vi "main.vi"() -> ()   [LabVIEW 2023]
uses:
  CONTROLS/states.ctl
panel:
  out "Meldung":string
  out "Enum":T1
  in  "stop":bool
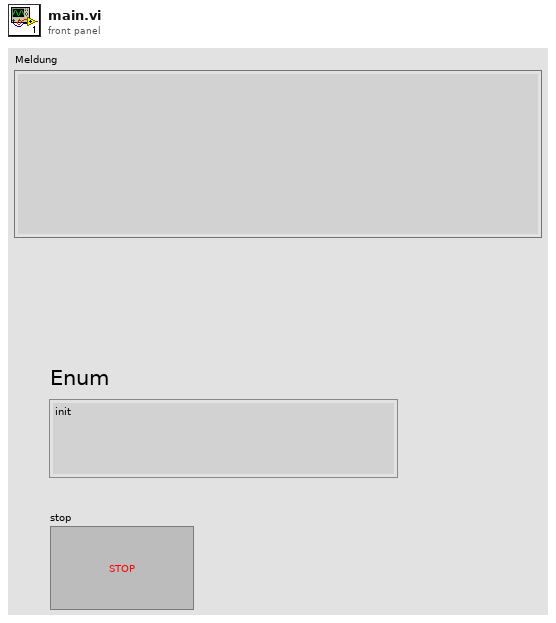
[diagram p1: front panel]
types:
  T1 = typedef "states.ctl" = enum16{"init", "read", "write", "Kundeneingabe", "Betonauswahl", "Bezahlprozeß", "Rechnung", "Zudaten mit Gewichtmessung", "Stop"}
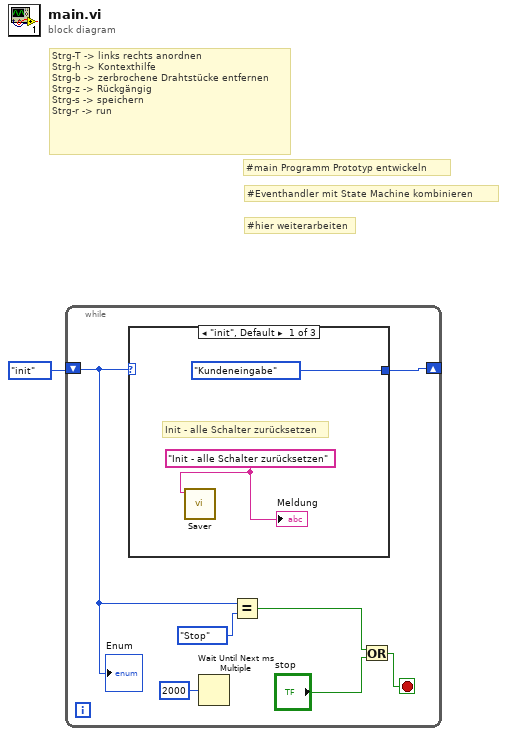
[diagram p0: block diagram]
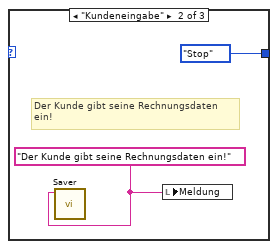
[diagram p2: hidden frame]
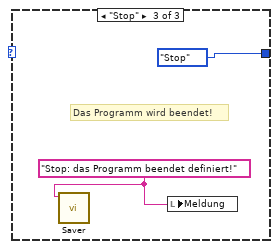
[diagram p3: hidden frame]
diagram:
  # "#hier weiterarbeiten"
  # "#Eventhandler mit State Machine kombinieren"
  # "#main Programm Prototyp entwickeln"
  # "Strg-T -> links rechts anordnen\nStrg-h -> Kontexthilfe\nStrg-b -> zerbrochene Drahtstücke entfernen\nStrg-z -> Rückgängig\nStrg-s -> speichern\nStrg-r -> run"
  n1 = while {
    shift-right: [w8] -> _
    shift-left: states."init" -> [w6]
    stop <- w3 stop-if-true
    n2 = case shown="\"init\", Default" w6 {
      tunnel: [states."Kundeneingabe" states."Stop" states."Stop"] -> w8
      frame "init", Default {
        w9 = "Init - alle Schalter zurücksetzen" ("Meldung")
        # "Init - alle Schalter zurücksetzen"
        n3 = call "Saver.vi"("TEXT"=w9) -> ()  [unwired: 10 in, 1 out]
        "Meldung" <- w9
      }
      frame "Kundeneingabe" {
        w11 = "Der Kunde gibt seine Rechnungsdaten ein!" ("Meldung")
        # "Der Kunde gibt seine Rechnungsdaten \nein!"
        n4 = call "Saver.vi"("TEXT"=w11) -> ()  [unwired: 10 in, 1 out]
        n5 = local write "Meldung"(w11) -> ()
      }
      frame "Stop" {
        w13 = "Stop: das Programm beendet definiert!" ("Meldung")
        # "Das Programm wird beendet!"
        n6 = call "Saver.vi"("TEXT"=w13) -> ()  [unwired: 10 in, 1 out]
        n7 = local write "Meldung"(w13) -> ()
      }
    }
    n8 = Wait Until Next ms Multiple(millisecond multiple=u32 2000) -> ()  [unwired: 1 out]
    n9 = Equal?(x=w6, y=states."Stop") -> (x = y?=w5:bool)
    n10 = Or(x=w5, y="stop") -> (x .or. y?=w3:bool)
    "Enum" <- w6
  }
